vi "Untitled 1.vi"   [LabVIEW 2014]
uses:
  <vilib>/measure/maspectr.llb/FFT Spectrum (Mag-Phase) for 1 Chan.vi
  <vilib>/measure/NI_MAPro.lvlib
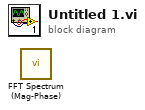
[diagram p0: block diagram]
diagram:
  n1 = call-poly <vilib>:"FFT Spectrum (Mag-Phase).vi"() -> ()  [unwired: 7 in, 5 out]
